vi "StopMotion.vi"(8 "error in (no error)":errorcluster, 11 "Picomoto8742ControllerClass in":refnum<class "Picomoto8742ControllerClass.lvclass">) -> (0 "error out":errorcluster, 3 "Picomoto8742ControllerClass out":refnum<class "Picomoto8742ControllerClass.lvclass">)   [LabVIEW 2020, in "Picomoto8742ControllerClass.lvclass"]
doc: "Send a STOP command to the physical device"
uses:
  Picomoto8742ControllerClass.lvclass
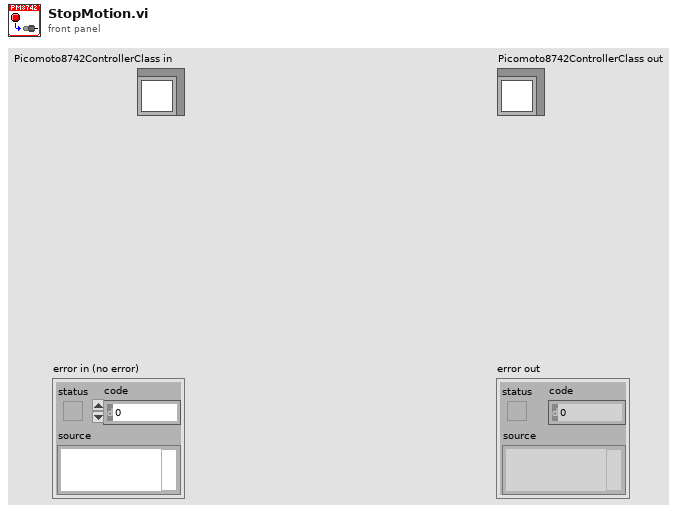
[diagram p1: front panel]
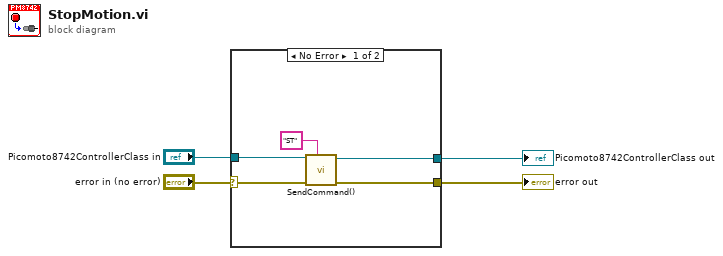
[diagram p0: block diagram]
diagram:
  n1 = case shown="No Error" "error in (no error)" {
    selector: "error in (no error)" -> [w9 w11]
    tunnel: [w6 w11] -> w3
    tunnel: [w5 w10] -> w1
    tunnel: "Picomoto8742ControllerClass in" -> [w8 w10]
    frame No Error {
      n2 = call "SendCommand().vi"("CMD"="ST" ("string"), "error in (no error)"=w9, "Picomoto8742ControllerClass in"=w8) -> ("error out"=w6:errorcluster, "Picomoto8742ControllerClass Out"=w5:refnum<class "Picomoto8742ControllerClass.lvclass">)  [unwired: 7 in]
    }
    frame Error {
    }
  }
  "error out" <- w3
  "Picomoto8742ControllerClass out" <- w1
